vi "PeriodicFilter-Format L3 Info String.vi"() -> (3 "Array":string[](array[string]))   [LabVIEW 2017, in "Communicable State Machine.lvlib"]
uses:
  Communicable State Machine.lvlib
  _Support/GlobalEvent/global-GEvnt Filter Change Flag.vi
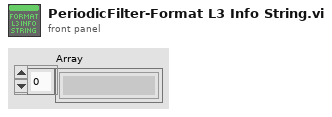
[diagram p1: front panel]
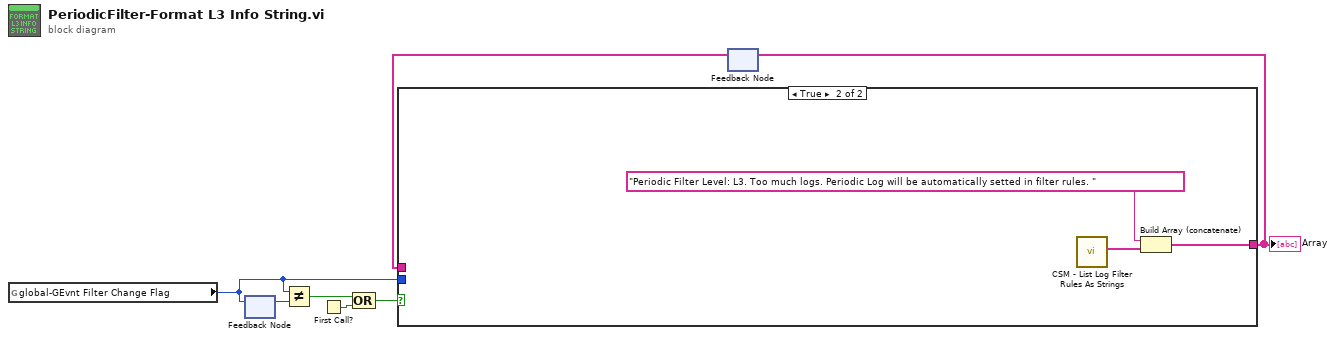
[diagram p0: block diagram]
diagram:
  n1 = global read "global-GEvnt Filter Change Flag.vi" "global-GEvnt Filter Change Flag"() -> (w1:u64)
  n2 = feedback #1() -> (w4:u64)  [unwired: 1 in]
  n3 = feedback-in #1(w1) -> ()
  n4 = Not Equal?(x=w1, y=w4) -> (x != y?=w5:bool)
  n5 = First Call?() -> (First Call?: T/F=w6:bool)
  n6 = Compound Arithmetic op=OR(w5, w6) -> (w3:bool)
  n7 = feedback #2() -> (w7:string[])  [unwired: 1 in]
  n8 = case shown="True" w3 {
    tunnel: [w8 w11] -> w2
    tunnel: w1 -> [_ _]
    tunnel: w7 -> [w8 _]
    frame False {
    }
    frame True {
      n9 = call "CSM - List Log Filter Rules As Strings.vi"() -> ("Rule Strings"=w9:string[])  [unwired: 10 in, 1 out]
      n10 = Build Array (concatenate)("Periodic Filter Level: L3. Too much logs. Periodic Log will be automatically setted in filter rules. " ("format string"), w9) -> (w11:string[])
    }
  }
  "Array" <- w2
  n11 = feedback-in #2(w2) -> ()
